vi "Get Bined Average.vi"(8 "error in (no error)":errorcluster, 11 "Bin Average in":refnum<class "Bin Average.lvclass">) -> (0 "error out":errorcluster, 1 "Binned average":dbl[][](array[numeric]), 2 "X ref array":dbl[](array[numeric]), 3 "Bin Average out":refnum<class "Bin Average.lvclass">)   [LabVIEW 2016, in "Bin Average.lvclass"]
uses:
  Bin Average.lvclass
  Bin Average.lvclass/Bin Average.ctl
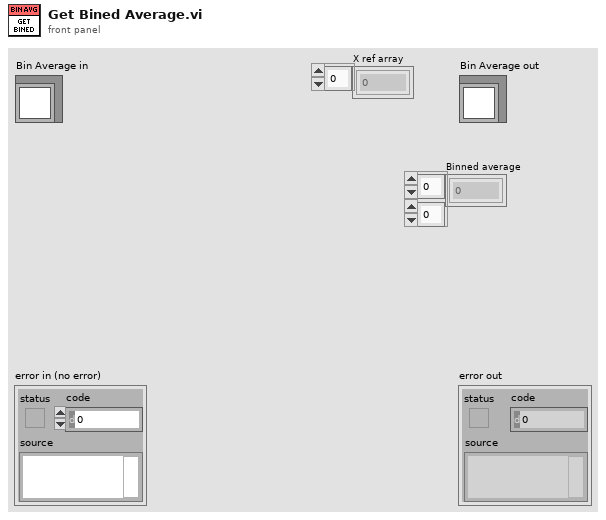
[diagram p1: front panel]
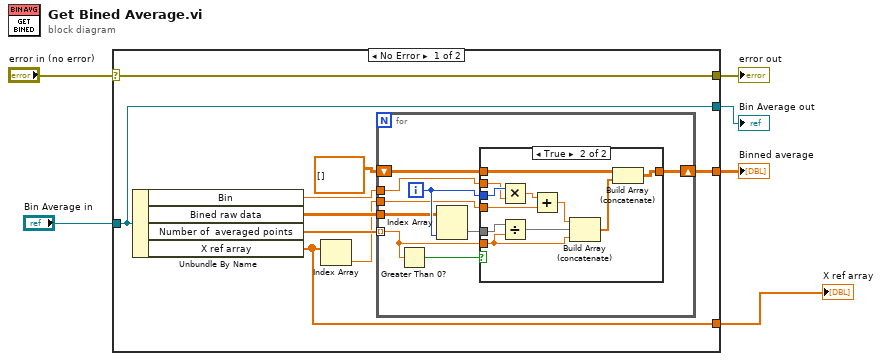
[diagram p0: block diagram]
diagram:
  n1 = case shown="No Error" "error in (no error)" {
    selector: "error in (no error)" -> [w15 w38]
    tunnel: [w15 w38] -> w5
    tunnel: [w14 w37] -> w3
    tunnel: "Bin Average in" -> [w14 w37]
    tunnel: [w8 _] -> w2
    tunnel: [w7 _] -> w1
    frame No Error {
      n2 = Unbundle By Name(w14) -> ("Bin"=w12:dbl, "Bined raw data"=w11:dbl[][], "Number of  averaged points"=w10:dbl[], "X ref array"=w7:dbl[])
      n3 = Index Array(array=w7) -> (element=w9:dbl)  [unwired: 1 in]
      n4 = for {
        tunnel: w10 -> [w16] mode=indexing
        tunnel: w12 -> [w22]
        tunnel: w9 -> [w21]
        shift-right: [w19] -> w8
        shift-left: dbl[][] [] -> [w18]
        tunnel: w11 -> [w20]
        i -> [w23]
        n5 = Greater Than 0?(x=w16) -> (x > 0?=w17:bool)
        n6 = Index Array(array=w20, index (col)=w23) -> (element=w24:dbl[])  [unwired: 1 in]
        n7 = case shown="True" w17 {
          tunnel: w24 -> [_ w36]
          tunnel: w23 -> [_ w35]
          tunnel: w22 -> [_ w34]
          tunnel: w21 -> [_ w33]
          tunnel: w16 -> [_ w29]
          tunnel: [w25 w28] -> w19
          tunnel: w18 -> [w25 w26]
          frame False {
          }
          frame True {
            n8 = Multiply(x=w35, y=w34) -> (x*y=w32:dbl)
            n9 = Divide(x=w36, y=w29) -> (x/y=w30:dbl[])
            n10 = Add(x=w32, y=w33) -> (x+y=w31:dbl)
            n11 = Build Array (concatenate)(w31, w30, w29) -> (w27:dbl[])
            n12 = Build Array (concatenate)(w26, w27) -> (w28:dbl[][])
          }
        }
      }
    }
    frame Error {
    }
  }
  "error out" <- w5
  "Bin Average out" <- w3
  "Binned average" <- w2
  "X ref array" <- w1
